vi "PID-Parameter Druckregler SysLog.vi"(11 "New Values":T1[][](array[typedef]) format="%#_5g") -> ()   [LabVIEW 2020, in "Erweiterte Konfig.lvlib"]
uses:
  Erweiterte Konfig.lvlib
  Visualisierungs Elemente/Zahlen-Eingabefeld.ctl
  cRIO/PC/Aktionen FGV Druckregler.ctl
  SysLog/SysLog Interface.ctl
  cRIO/PC/Kommunikation mit cRIO.lvlib
  SysLog/SysLog.lvlib
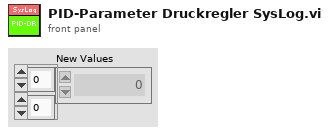
[diagram p1: front panel]
types:
  T1 = typedef "Zahlen-Eingabefeld.ctl" = sgl
  T2 = typedef "Kommunikation mit cRIO.lvlib/Aktionen FGV Druckregler.ctl" = enum16{"lesen", "Parameter", "Istwerte"}
  T3 = typedef "SysLog.lvlib/SysLog Interface.ctl" = cluster{"Fehlermeldung":string, "Erfolgsmeldung":string, "Anzeige":bool, "SysLogIcon":enum16{"OK", "Warnung", "Fehler"}, "intern":bool}
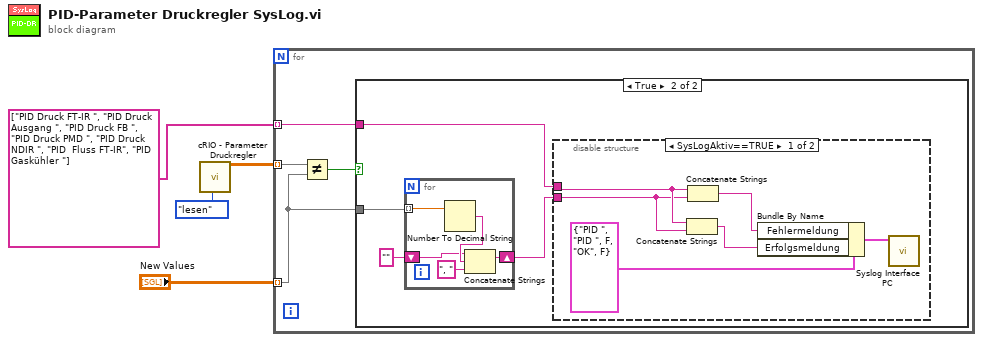
[diagram p0: block diagram]
diagram:
  n1 = call "cRIO - Parameter Druckregler.vi"("Aktion"=Aktionen_FGV_Druckregler."lesen") -> ("Parameter Regler"=w2:sgl[][])  [unwired: 9 in, 9 out]
  n2 = for {
    tunnel: "New Values" -> [w6] mode=indexing
    tunnel: w2 -> [w8] mode=indexing
    tunnel: string[] ["PID Druck FT-IR ", "PID Druck Ausgang ", "PID Druck FB ", "PID Druck PMD ", "PID Druck NDIR ", "PID  Fluss FT-IR", "PID Gaskühler "] -> [w5] mode=indexing
    n3 = Not Equal?(x=w8, y=w6) -> (x != y?=w7:bool)
    n4 = case shown="True" w7 {
      tunnel: w6 -> [_ w11]
      tunnel: w5 -> [_ w9]
      frame False {
      }
      frame True {
        n5 = for {
          tunnel: w11 -> [w23] mode=indexing
          shift-right: [w20] -> w10
          shift-left: "" -> [w21]
          n6 = Number To Decimal String(number=w23) -> (decimal integer string=w22:string)  [unwired: 1 in]
          n7 = Concatenate Strings(w21, w22, ", " ("String")) -> (w20:string)
        }
        n8 = disable-structure shown="SysLogAktiv==TRUE" {
          disable-tunnel: w9 -> [w14 _]
          disable-tunnel: w10 -> [w13 _]
          frame condition #0 (active) {
            n9 = Concatenate Strings(w14, w13) -> (w15:string)
            n10 = Concatenate Strings(w14, w13) -> (w16:string)
            n11 = Bundle By Name(cluster=T3 {"Fehlermeldung"="PID ", "Erfolgsmeldung"="PID ", "Anzeige"=FALSE, "SysLogIcon"=enum."OK", "intern"=FALSE} ("Cluster (in)"), "Fehlermeldung"=w16, "Erfolgsmeldung"=w15) -> (w17:T3)
            n12 = call "Syslog Interface PC.vi"("Cluster (in)"=w17) -> ()  [unwired: 10 in, 1 out]
          }
          frame condition #1 {
          }
        }
      }
    }
  }
